vi "Data_Changed-Boolean.vi"(1 "Data":bool=TRUE) -> (0 "Value Changed":bool)   [LabVIEW 2012]
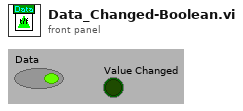
[diagram p1: front panel]
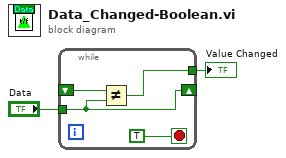
[diagram p0: block diagram]
diagram:
  n1 = while {
    shift-right: [w3] -> _
    shift-left: _ -> [w5]
    tunnel: "Data" -> [w3]
    tunnel: [w4] -> w2
    stop <- TRUE stop-if-true
    n2 = Not Equal?(x=w5, y=w3) -> (x != y?=w4:bool)
  }
  "Value Changed" <- w2
